vi "Read Non-Sequential Address (CMD-ONLY).vi"(7 "Target (1-8)":u8, 8 "error in (no error)":errorcluster, 10 "Address":u16 format="%04x", 11 "FPGA Interface in":refnum<class "FPGA Interface.lvclass">) -> (0 "error out":errorcluster)   [LabVIEW 2020, in "BCI-1553 API.lvlib" / "FPGA Interface.lvlib" / "FPGA Interface.lvclass"]
doc: "Reads an arbitrary address from a component in the 1553 Session. This method does not block and will not wait for data to return from the specified component."
uses:
  FPGA Interface.lvclass
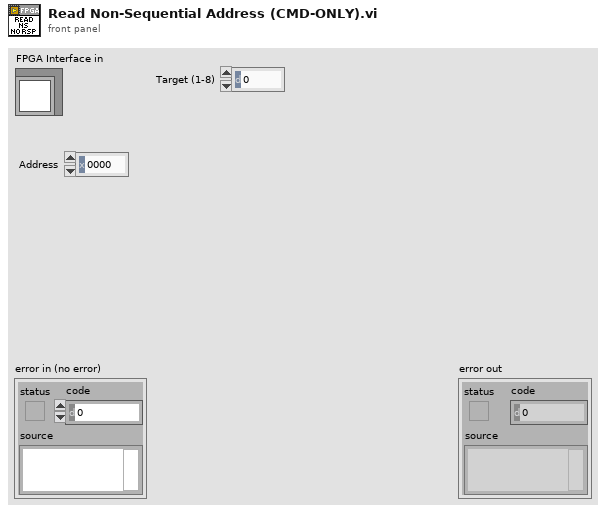
[diagram p1: front panel]
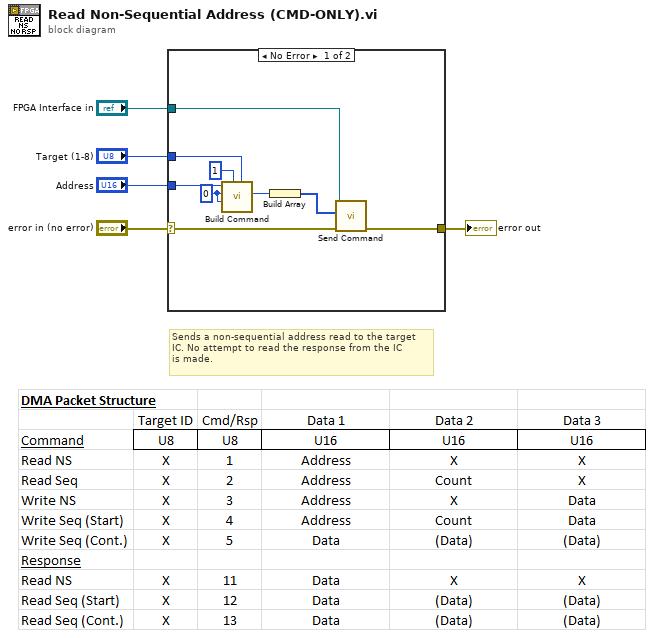
[diagram p0: block diagram]
diagram:
  # "Sends a non-sequential address read to the target\nIC. No attempt to read the response from the IC\nis made."
  n1 = case shown="No Error" "error in (no error)" {
    selector: "error in (no error)" -> [w11 w15]
    tunnel: [w9 w15] -> w4
    tunnel: "FPGA Interface in" -> [w10 _]
    tunnel: "Target (1-8)" -> [w8 _]
    tunnel: "Address" -> [w14 _]
    frame No Error {
      w6 = u16 0 ("Data 2")
      n2 = call "Build Command.vi"("Target"=w8, "CMD ID"=u8 1, "Data 3"=w6, "Data 2"=w6, "Data 1"=w14) -> ("Command"=w13:u64)  [unwired: 5 in, 1 out]
      n3 = Build Array(w13) -> (w12:u64[])
      n4 = call "Send Command.vi"("error in (no error)"=w11, "Data"=w12, "FPGA Interface in"=w10) -> ("error out"=w9:errorcluster)  [unwired: 8 in]
    }
    frame Error {
    }
  }
  "error out" <- w4
